vi "Stage3.vi"(0 "Start":bool, 1 "Stop":bool, 2 "Reset":bool, 3 "C":bool[][](array[boolean]), 4 "Stage table":u32[][](array[numeric])=[[0, 2, 2, 2, 2], [0, 3, 3, 3, 3], [0, 4, 4, 4, 4], [0, 0, 0, 0, 0]], 6 "Step":bool, 7 "End step":u32, 9 "Descriptions":string[](array[string])) -> (13 "Description":string, 14 "Start":bool, 15 "Stop":bool, 16 "End":bool, 17 "t":u32, 18 "N curr":u32)   [LabVIEW 2019]
uses:
  Logik/Logik.lvlib
  Trigers/Triggers.lvlib
  Timer Delay/Timers.lvlib
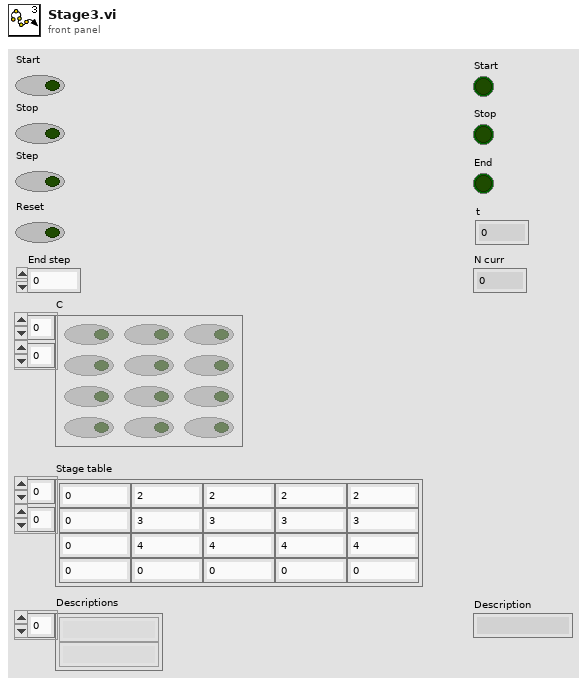
[diagram p1: front panel]
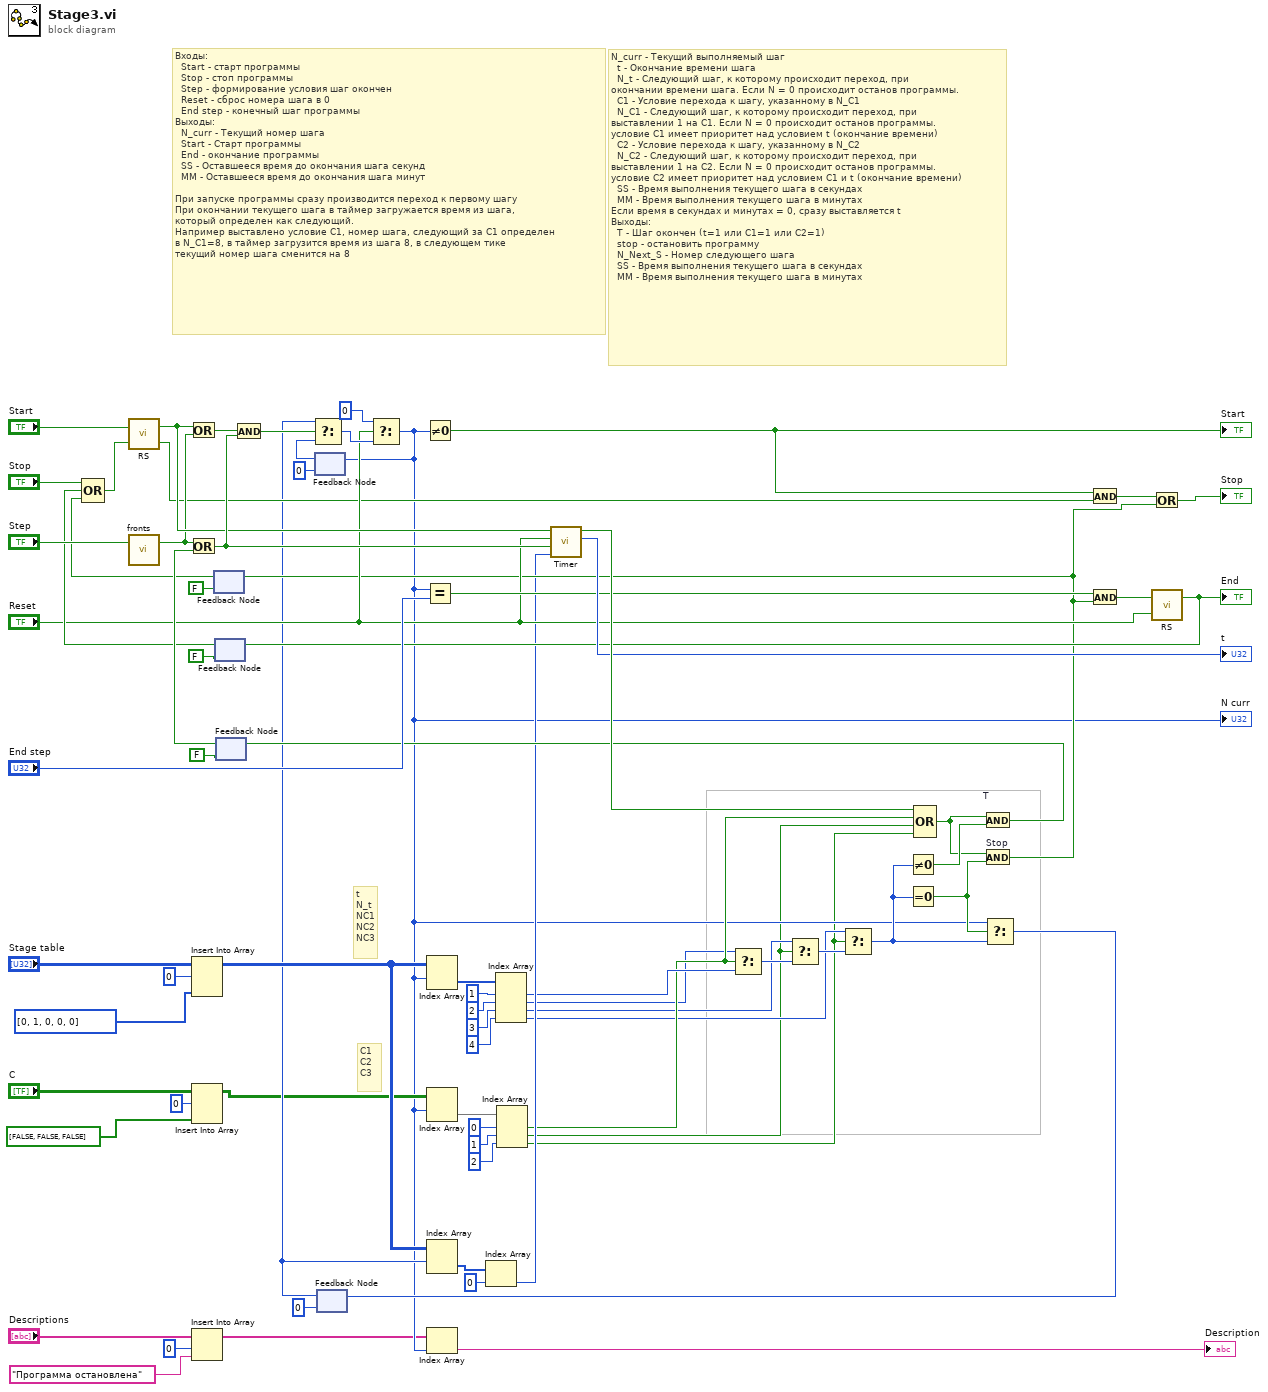
[diagram p0: block diagram]
diagram:
  # "C1\nC2\nC3"
  # "t\nN_t\nNC1\nNC2\nNC3"
  # "N_curr - Текущий выполняемый шаг\n  t - Окончание времени шага\n  N_t - Следующий шаг, к которому происходит переход, при\nокончании времени шага. Если N = 0 происходит останов программы.\n  C1 - Условие перехода к шагу, указанному в N_C1\n  N_C1 - Следующий шаг, к которому происходит переход, при\nвыставлении 1 на С1. Если N = 0 происходит останов программы.\nусловие С1 имеет приоритет над условием t (окончание времени)\n  C2 - Условие перехода к шагу, указанному в N_C2\n  N_C2 - Следующий шаг, к которому происходит переход, при\nвыставлении 1 на С2. Если N = 0 происходит останов программы.\nусловие С2 имеет приоритет над условием С1 и t (окончание времени)\n  SS - Время выполнения текущего шага в секундах\n  MM - Время выполнения текущего шага в минутах\nЕсли время в секундах и минутах = 0, сразу выставляется t\nВыходы:\n  T - Шаг окончен (t=1 или C1=1 или С2=1)\n  stop - остановить программу\n  N_Next_S - Номер следующего шага\n  SS - Время выполнения текущего шага в секундах\n  MM - Время выполнения текущего шага в минутах"
  # "Входы:\n  Start - старт программы\n  Stop - стоп программы\n  Step - формирование условия шаг окончен\n  Reset - сброс номера шага в 0\n  End step - конечный шаг программы\nВыходы:\n  N_curr - Текущий номер шага\n  Start - Старт программы\n  End - окончание программы\n  SS - Оставшееся время до окончания шага секунд\n  MM - Оставшееся время до окончания шага минут\n\nПри запуске программы сразу производится переход к первому шагу\nПри окончании текущего шага в таймер загружается время из шага,\nкоторый определен как следующий.\nНапример выставлено условие C1, номер шага, следующий за С1 определен\nв N_C1=8, в таймер загрузится время из шага 8, в следующем тике \nтекущий номер шага сменится на 8"
  n1 = call "fronts.vi"("in"="Step") -> ("raise"=w63:bool)  [unwired: 1 in, 1 out]
  n2 = Insert Into Array(array="Stage table", index (row)=0 ("index"), new element=u32[] [0, 1, 0, 0, 0]) -> (w48:u32[][])  [unwired: 1 in]
  n3 = Insert Into Array(array="C", index (row)=0, new element=bool[] [FALSE, FALSE, FALSE]) -> (w20:bool[][])  [unwired: 1 in]
  n4 = Insert Into Array(array="Descriptions", index=0, new element="Программа остановлена" ("new element/subarray")) -> (w11:string[])
  n5 = feedback #1(FALSE ("Q")) -> (w53:bool)
  n6 = feedback #2(FALSE ("Q")) -> (w52:bool)
  n7 = Compound Arithmetic op=OR("Stop", w52, w53) -> (w72:bool)
  n8 = call "RS.vi"("R"=w72, "S"="Start") -> ("~Q"=w37:bool, "Q"=w65:bool)
  n9 = Or(x=w65, y=w63) -> (x .or. y?=w74:bool)
  n10 = feedback #3(FALSE ("Q")) -> (w55:bool)
  n11 = Or(x=w63, y=w55) -> (x .or. y?=w66:bool)
  n12 = And(x=w74, y=w66) -> (x .and. y?=w73:bool)
  n13 = feedback #4(u32 0) -> (w45:u32)
  n14 = feedback #5(u32 0) -> (w30:u32)
  n15 = Select(t=w30, s=w73, f=w45) -> (s? t:f=w47:u32)
  n16 = Select(t=u32 0, s="Reset", f=w47) -> (s? t:f=w15:u32)
  "N curr" <- w15
  n17 = feedback-in #4(w15) -> ()
  n18 = Not Equal To 0?(x=w15) -> (x != 0?=w43:bool)
  "Start" <- w43
  n19 = Equal?(x=w15, y="End step") -> (x = y?=w40:bool)
  n20 = Index Array(array=w48, index (row)=w15) -> (element=w24:u32[])  [unwired: 1 in]
  n21 = Index Array(array=w20, index (row)=w15) -> (element=w19:bool[])  [unwired: 1 in]
  n22 = Index Array(array=w48, index (row)=w30) -> (element=w28:u32[])  [unwired: 1 in]
  n23 = Index Array(array=w11, index=w15) -> (element=→"Description":string)
  n24 = Index Array(array=w28, index=0) -> (element=w27:u32)
  n25 = Index Array(array=w24, index #1=1 ("index"), index #2=2 ("index"), index #3=3 ("index"), index #4=4 ("index")) -> (element #1=w25:u32, element #2=w10:u32, element #3=w8:u32, element #4=w6:u32)
  n26 = Index Array(array=w19, index #1=0 ("index"), index #2=1 ("index"), index #3=2 ("index")) -> (element #1=w17:bool, element #2=w4:bool, element #3=w3:bool)
  n27 = call "Timer.vi"("ms"=w27, "Load (F)"=w66, "Reset (F)"="Reset", "Start (T)"=w65) -> ("t ms"=→"t":u32, "End"=w58:bool)  [unwired: 5 in]
  n28 = Select(t=w10, s=w17, f=w25) -> (s? t:f=w62:u32)
  n29 = Select(t=w8, s=w4, f=w62) -> (s? t:f=w35:u32)
  n30 = Select(t=w6, s=w3, f=w35) -> (s? t:f=w34:u32)
  n31 = Not Equal To 0?(x=w34) -> (x != 0?=w61:bool)
  n32 = Equal To 0?(x=w34) -> (x = 0?=w59:bool)
  n33 = Compound Arithmetic op=OR(w58, w17, w4, w3) -> (w60:bool)
  n34 = And "T"(x=w60, y=w61) -> (x .and. y?=w56:bool)
  n35 = feedback-in #3(w56) -> ()
  n36 = And "Stop"(x=w60, y=w59) -> (x .and. y?=w36:bool)
  n37 = feedback-in #1(w36) -> ()
  n38 = Select(t=w15, s=w59, f=w34) -> (s? t:f=w49:u32)
  n39 = feedback-in #5(w49) -> ()
  n40 = And(x=w43, y=w37) -> (x .and. y?=w39:bool)
  n41 = And(x=w40, y=w36) -> (x .and. y?=w68:bool)
  n42 = Or(x=w39, y=w36) -> (x .or. y?=→"Stop":bool)
  n43 = call "RS.vi"("R"="Reset", "S"=w68) -> ("Q"=w41:bool)  [unwired: 1 out]
  "End" <- w41
  n44 = feedback-in #2(w41) -> ()
